vi "PH_Tektronix_7000.set Cursor Deltas.vi"(0 "i ref in":refnum<vi>, 5 "error in (no eror)":errorcluster) -> (14 "i ref out":refnum<vi>, 19 "error out":errorcluster)   [LabVIEW 2014, in "PH_Tektronix_7000.lvlib"]
doc: "This VI calculates the difference of the cursor position and sets the value to the related GUI elements."
uses:
  PH_Tektronix_7000.lvlib
  PH_Basics/PH_Common/PH_Common.lvlib
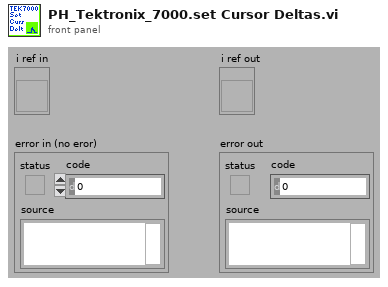
[diagram p1: front panel]
types:
  T1 = typedef "PH_Tektronix_7000.lvlib/PH_Tektronix_7000.i attribute.ctl" = cluster{"VISA Resource Name":refnum<visa-resource-name>, "IDN":cluster{"Instrument Driver":string, "Instrument Firmware":string, "Model":string, "Serial Number":string}, "Selftest":cluster{"Result":i32, "Message":string}, "Trigger Configuration":T2, "Acquisition Configuration":T3, "GUI Refs":T4, "State":T5, "Error Message":string, "Allow Prdc Loop?":bool, "Channel 1":T6, "Channel 2":T6, "Channel 3":T6, "Channel 4":T6, "Data CH 1":waveform(dbl), "Data CH 2":waveform(dbl), "Data CH 3":waveform(dbl), "Data CH 4":waveform(dbl), "Allow config?":bool, "Name Channel 1":string, "Name Channel 2":string, "Name Channel 3":string, "Name Channel 4":string, "Fetch Data before sending to PSDB?":bool, "Constructor passed?":bool, "Data taken at":timestamp, "Plot Colors":u32[], "Default VISA Resource":string}
  T2 = typedef "PH_Tektronix_7000.lvlib/PH_Tektronix_7000.Trigger Config.ctl" = cluster{"Source":u16, "Level [V]":dbl, "Slope":u16, "Coupling":u16, "Trigger Mode":u16}
  T3 = typedef "PH_Tektronix_7000.lvlib/PH_Tektronix_7000.Acquisition Config.ctl" = cluster{"Record Length":u32, "Timebase [s/div]":dbl, "Position [%]":dbl, "Acquisition Type":u16, "Average Waveforms":i32, "Envelope Waveforms":i32, "WfmDB Samples":i32, "Continuous?":bool, "Delay [s]":dbl, "Run?":bool}
  T4 = typedef "PH_Tektronix_7000.lvlib/PH_Tektronix_7000.GUI Refs.ctl" = cluster{"Graph":refnum<vi>, "State":refnum<vi>, "Delete":refnum<vi>, "VISA Resource":refnum<vi>, "Allow Configure":refnum<vi>, "Fetch Data":refnum<vi>, "Fetch before sending Data to PSDB":refnum<vi>, "Name Channel 1":refnum<vi>, "Name Channel 2":refnum<vi>, "Name Channel 3":refnum<vi>, "Name Channel 4":refnum<vi>, "Prdc Intervall [ms]":refnum<vi>, "Data taken":refnum<vi>, "Model":refnum<vi>, "Serial Number":refnum<vi>, "Firmware":refnum<vi>, "Driver":refnum<vi>, "Acquisition":refnum<vi>, "Trigger":refnum<vi>, "Cursor: D Time [s]":refnum<vi>, "Cursor: D Signal [V]":refnum<vi>, "Channel 1":refnum<vi>, "Channel 2":refnum<vi>, "Channel 3":refnum<vi>, "Channel 4":refnum<vi>}
  T5 = typedef "PH_StatusHandler.lvlib/PH_StatusHandler.Status.ctl" = i16
  T6 = typedef "PH_Tektronix_7000.lvlib/PH_Tektronix_7000.Channel Config.ctl" = cluster{"Enable Channel":bool, "Bandwidth":u16, "Input Impedance":u16, "Vertical Coupling":u16, "Probe Attenuation":dbl, "Range [V/div]":dbl, "Position [div]":dbl, "Bandwidth raw":string}
  T7 = typedef "LVCursorListTypeDef.ctl" = cluster{"Name":string, "Color":u32, "Style":u8, "Point Style":u8, "Name Visible":bool, "Allow Drag":bool, "Cursor Mode":u32, "Plot":i32, "Index":i32, "Position":cluster{"X":dbl, "Y":dbl}, "X Scale":u32, "Y Scale":u32, "Watch Plots":i32[], "Watch All Plots":bool, "Plot Area":i32, "Label Offset":cluster{"X":dbl, "Y":dbl}}[]
  T8 = cluster{"Name":string, "Color":u32, "Style":u8, "Point Style":u8, "Name Visible":bool, "Allow Drag":bool, "Cursor Mode":u32, "Plot":i32, "Index":i32, "Position":cluster{"X":dbl, "Y":dbl}, "X Scale":u32, "Y Scale":u32, "Watch Plots":i32[], "Watch All Plots":bool, "Plot Area":i32, "Label Offset":cluster{"X":dbl, "Y":dbl}}
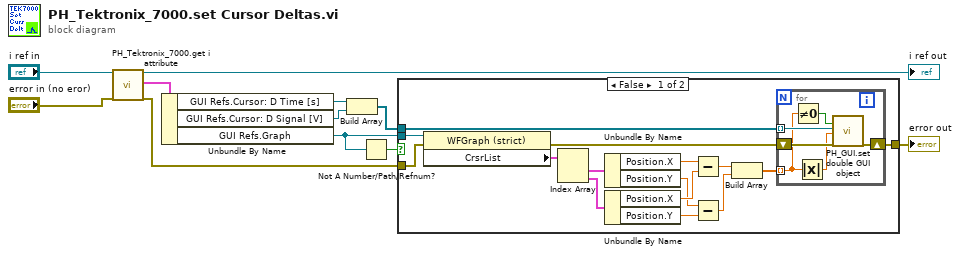
[diagram p0: block diagram]
diagram:
  n1 = call "PH_Tektronix_7000.get i attribute.vi"("i ref in"="i ref in", "error in (no error)"="error in (no eror)") -> ("i ref out"=→"i ref out":refnum<vi>, "i attribute"=w8:T1, "error out"=w4:errorcluster)  [unwired: 15 in]
  n2 = Unbundle By Name(w8) -> ("GUI Refs.Cursor: D Time [s]"=w7:refnum<vi>, "GUI Refs.Cursor: D Signal [V]"=w6:refnum<vi>, "GUI Refs.Graph"=w2:refnum<vi>)
  n3 = Build Array(w7, w6) -> (w5:refnum<vi>[])
  n4 = Not A Number/Path/Refnum?(number/path/refnum=w2) -> (NaN/Path/Refnum?=w3:bool)
  n5 = case shown="False" w3 {
    tunnel: w2 -> [w26 _]
    tunnel: [w15 w33] -> w1
    tunnel: w5 -> [w13 _]
    tunnel: w4 -> [w12 w33]
    frame False {
      n6 = property class="WFGraph (strict)"(reference=w26, error in=w12) -> (error out=w16:errorcluster, "CrsrList"=w25:T7)  [unwired: 1 out]
      n7 = Index Array(array=w25) -> (element #1=w24:T8, element #2=w23:T8)  [unwired: 2 in]
      n8 = Unbundle By Name(w24) -> ("Position.X"=w22:dbl, "Position.Y"=w19:dbl)
      n9 = Unbundle By Name(w23) -> ("Position.X"=w21:dbl, "Position.Y"=w20:dbl)
      n10 = Subtract(x=w22, y=w21) -> (x-y=w18:dbl)
      n11 = Subtract(x=w19, y=w20) -> (x-y=w17:dbl)
      n12 = Build Array(w18, w17) -> (w14:dbl[])
      n13 = for {
        shift-right: [w31] -> w15
        shift-left: w16 -> [w32]
        tunnel: w13 -> [w30] mode=indexing
        tunnel: w14 -> [w28] mode=indexing
        n14 = Not Equal To 0?(x=w28) -> (x != 0?=w29:bool)
        n15 = Absolute Value(x=w28) -> (abs(x)=w27:dbl)
        n16 = call "PH_GUI.set double GUI object.vi"("visible (true)"=w29, "GUI object Ref"=w30, "value"=w27, "error in (no error)"=w32) -> ("error out"=w31:errorcluster)  [unwired: 15 in]
      }
    }
    frame True {
    }
  }
  "error out" <- w1
